vi "Test Get Class Instance.vi"(8 "error in (no error)":errorcluster, 11 "TestCase in":refnum<class "Test FP.lvclass">) -> (0 "error out":errorcluster, 3 "TestCase out":refnum<class "Test FP.lvclass">)   [LabVIEW 2020, in "Test FP.lvclass"]
uses:
  Test FP.lvclass
  d5a3454a-fa88-4a14-bf58-25560348bcbd.vi
  <vilib>/Comparison/Equal/Equal Functor/Equal Functor.lvclass
  <vilib>/addons/_JKI Toolkits/VI Tester/TestCase.llb/TestCase.lvclass
  C:/Program Files (x86)/National Instruments/LabVIEW 2020/vi.lib/addons/_JKI Toolkits/VI Tester/TestCase.llb/TestCase.lvclass
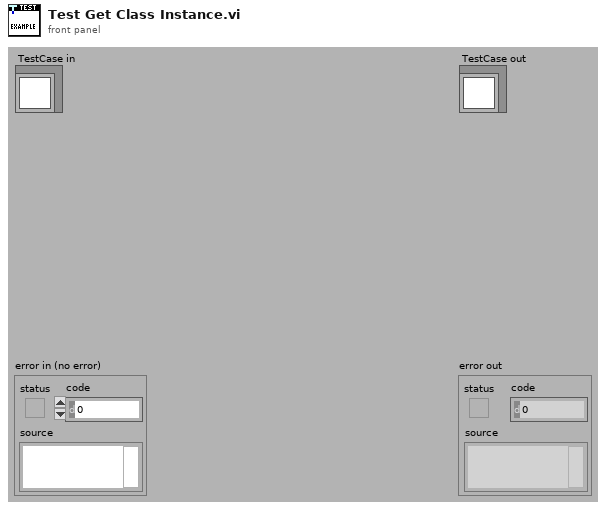
[diagram p1: front panel]
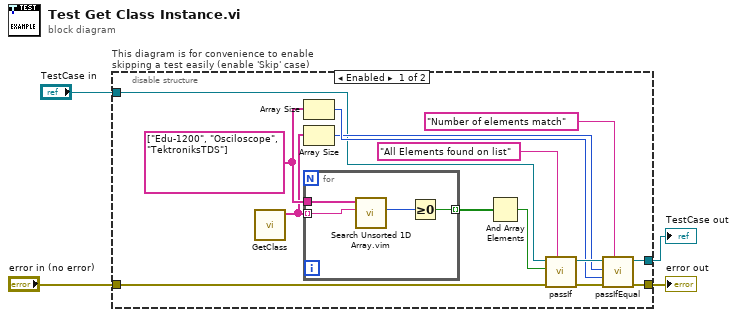
[diagram p0: block diagram]
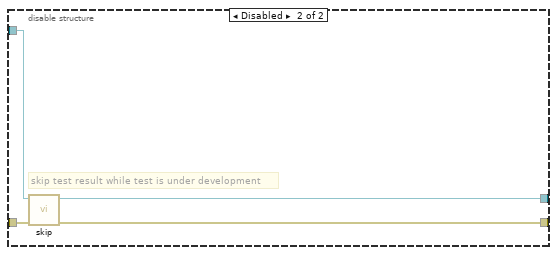
[diagram p2: hidden frame]
diagram:
  n1 = disable-structure "This diagram is for convenience to enable skipping a test easily (enable 'Skip' case)" shown="Enabled" {
    disable-tunnel: "TestCase in" -> [w8 w26]
    disable-tunnel: [w6 w24] -> w1
    disable-tunnel: [w7 w25] -> w3
    disable-tunnel: "error in (no error)" -> [w5 w23]
    frame Enabled {
      w10 = string[] ["Edu-1200", "Osciloscope", "TektroniksTDS"] ("Class Avaliables")
      n2 = call "GetClass.vi"() -> ("Class Avaliables"=w9:string[])  [unwired: 11 in]
      n3 = Array Size(array=w10) -> (size(s)=w15:i32)
      n4 = Array Size(array=w9) -> (size(s)=w14:i32)
      n5 = for {
        tunnel: w10 -> [w19]
        tunnel: w9 -> [w20] mode=indexing
        tunnel: [w22] -> w18 mode=indexing
        n6 = call "Search Unsorted 1D Array.vim"("element"=w20, "unsorted 1D array"=w19) -> ("index of element"=w21:i32)  [unwired: 9 in]
        n7 = Greater Or Equal To 0?(x=w21) -> (x >= 0?=w22:bool)
      }
      n8 = And Array Elements(Boolean array=w18) -> (logical AND=w13:bool)
      n9 = call-dynamic "passIf.vi"("custom report message (\"\")"="All Elements found on list" ("custom report message (\"\")"), "error in (no error)"=w5, "pass"=w13, "TestCase in"=w8) -> ("error out"=w16:errorcluster, "TestCase out"=w17:refnum<class "Test FP.lvclass">)  [unwired: 6 in]
      n10 = call-dynamic "passIfEqual.vi"("custom report message (\"\")"="Number of elements match" ("custom report message (\"\")"), "error in (no error)"=w16, "y"=w15, "x"=w14, "TestCase in"=w17) -> ("error out"=w7:errorcluster, "TestCase out"=w6:refnum<class "Test FP.lvclass">)  [unwired: 5 in]
    }
    frame Disabled {
      # "skip test result while test is under development"
      n11 = call <vilib>:"skip.vi"("error in (no error)"=w23, "TestCase in"=w26) -> ("error out"=w25:errorcluster, "TestCase out"=w24:refnum<class "Test FP.lvclass">)  [unwired: 8 in]
    }
  }
  "error out" <- w3
  "TestCase out" <- w1
